vi "setUp.vi"(8 "error in":errorcluster, 11 "reference in":refnum<class "Create Execution Unit.lvclass">) -> (0 "error out":errorcluster, 3 "reference out":refnum<class "Create Execution Unit.lvclass">)   [LabVIEW 2020, in "Create Execution Unit.lvclass"]
doc: "setUp runs prior to the test method during test execution. Use this method to initialize any object data required by your tests."
uses:
  Create Execution Unit.lvclass
  C:/Program Files (x86)/National Instruments/LabVIEW 2020/vi.lib/addons/_JKI Toolkits/VI Tester/TestCase.llb/TestCase.lvclass
  Create Execution Unit.lvclass/Create Execution Unit.ctl
  <vilib>/addons/_JKI Toolkits/VI Tester/TestCase.llb/TestCase.lvclass
  niveristand-custom-device-testing-tools/VeriStandScriptingTestCase/VeriStandScriptingTestCase.lvclass
  niveristand-custom-device-testing-tools/VeriStandTestUtilities/VeriStandTestUtilities.lvlib
  C:/Git/niveristand-custom-device-testing-tools/VeriStandScriptingTestCase/VeriStandScriptingTestCase.lvclass
  C:/Git/niveristand-ballard-milStd1553-custom-device/Source/Custom Device Support/Tests/Unit/Create Execution Unit/Create Execution Unit.lvclass
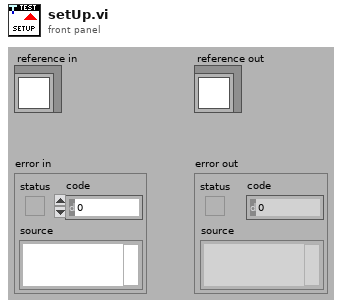
[diagram p1: front panel]
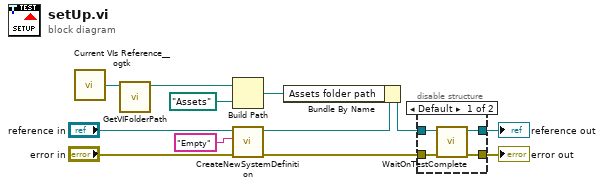
[diagram p0: block diagram]
diagram:
  n1 = call <userlib>:"Current VIs Reference__ogtk.vi"() -> ("Current VI's reference"=w6:refnum<vi>)  [unwired: 5 in]
  n2 = call "GetVIFolderPath.vi"("VI Reference in"=w6) -> ("VI Folder Path out"=w5:path)  [unwired: 9 in, 1 out]
  n3 = Build Path(base path=w5, name or relative path=path "Assets") -> (appended path=w3:path)
  n4 = call "CreateNewSystemDefinition.vi"("error in (no error)"="error in", "System Definition Name"="Empty", "VeriStandScriptingTestCase in"="reference in") -> ("error out"=w7:errorcluster, "VeriStandScriptingTestCase out"=w2:refnum<class "Create Execution Unit.lvclass">)  [unwired: 7 in]
  n5 = Bundle By Name(cluster=w2, "Assets folder path"=w3) -> (w1:refnum<class "Create Execution Unit.lvclass">)
  n6 = disable-structure shown="Default" {
    disable-tunnel: w7 -> [w16 w17]
    disable-tunnel: [w15 w17] -> w12
    disable-tunnel: [w14 w18] -> w11
    disable-tunnel: w1 -> [w13 w18]
    frame condition #0 (active) {
      n7 = call <vilib>:"WaitOnTestComplete.vi"("error in (no error)"=w16, "TestCase in"=w13) -> ("error out"=w15:errorcluster, "TestCase out"=w14:refnum<class "Create Execution Unit.lvclass">)  [unwired: 8 in]
    }
    frame condition #1 {
    }
  }
  "error out" <- w12
  "reference out" <- w11
